vi "ResetS0Bit.vi"(8 "error in (no error)":errorcluster, 9 "Address":u8, 10 "bitnumber":u32, 11 "board_sel":u32=1) -> (0 "error out":errorcluster)   [LabVIEW 2015, in "ESLSCDLL.lvlib"]
uses:
  ESLSCDLL.lvlib
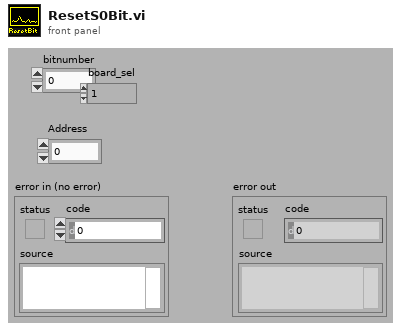
[diagram p1: front panel]
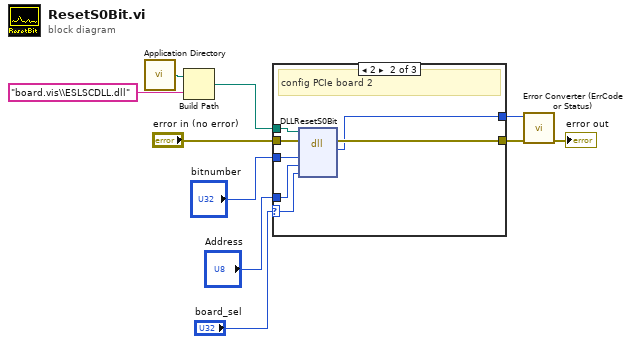
[diagram p0: block diagram]
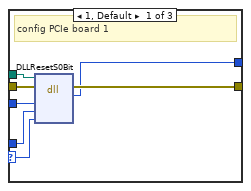
[diagram p2: hidden frame]
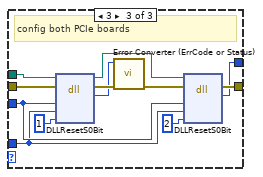
[diagram p3: hidden frame]
diagram:
  n1 = call <vilib>:"Application Directory.vi"() -> ("Application Directory"=w3:path)
  n2 = Build Path(base path=w3, name or relative path="board.vis\\ESLSCDLL.dll") -> (appended path=w1:path)
  n3 = case shown="2" "board_sel" {
    selector: "board_sel" -> [w17 w24 _]
    tunnel: "bitnumber" -> [w16 w23 w34]
    tunnel: "Address" -> [w15 w22 w33]
    tunnel: "error in (no error)" -> [w14 w21 w30]
    tunnel: [w13 w20 w28] -> w5
    tunnel: [w12 w19 w27] -> w4
    tunnel: w1 -> [w11 w18 w26]
    frame 1, Default {
      # "config PCIe board 1"
      n4 = dll-call lib="C:/ENTW/PCIE/LV64/board.vis/ESLSCDLL.dll" fn="DLLResetS0Bit" ("lwlscdll.dll:DLLRsTOREG")(path in=w11, error in=w14, "bitnumber"=w16, "Address"=w15, "drv"=w17) -> (error out=w13:errorcluster, "es_status_codes"=w12:i32)  [unwired: 4 in, 1 out]
    }
    frame 2 {
      # "config PCIe board 2"
      n5 = dll-call lib="C:/ENTW/PCIE/LV64/board.vis/ESLSCDLL.dll" fn="DLLResetS0Bit" ("lwlscdll.dll:DLLRsTOREG")(path in=w18, error in=w21, "bitnumber"=w23, "Address"=w22, "drv"=w24) -> (error out=w20:errorcluster, "es_status_codes"=w19:i32)  [unwired: 4 in, 1 out]
    }
    frame 3 {
      # "config both PCIe boards"
      n6 = dll-call lib="C:/ENTW/PCIE/LV64/board.vis/ESLSCDLL.dll" fn="DLLResetS0Bit" ("lwlscdll.dll:DLLRsTOREG")(path in=w26, error in=w30, "bitnumber"=w34, "Address"=w33, "drv"=u32 1) -> (path out=w25:path, error out=w32:errorcluster, "es_status_codes"=w31:i32)  [unwired: 4 in]
      n7 = call "Error Converter (ErrCode or Status).vi"("error in (no error)"=w32, "error code"=w31) -> ("error out"=w29:errorcluster)  [unwired: 9 in]
      n8 = dll-call lib="C:/ENTW/PCIE/LV64/board.vis/ESLSCDLL.dll" fn="DLLResetS0Bit" ("lwlscdll.dll:DLLRsTOREG")(path in=w25, error in=w29, "bitnumber"=w34, "Address"=w33, "drv"=u32 2) -> (error out=w28:errorcluster, "es_status_codes"=w27:i32)  [unwired: 4 in, 1 out]
    }
  }
  n9 = call "Error Converter (ErrCode or Status).vi"("error in (no error)"=w5, "error code"=w4) -> ("error out"=→"error out":errorcluster)  [unwired: 9 in]
